vi "Update Library.vi"(8 "error in":errorcluster, 10 "Library":refnum<class "Library.lvclass">, 11 "Project in":refnum<class "Project.lvclass">) -> (0 "error out":errorcluster, 3 "Project out":refnum<class "Project.lvclass">)   [LabVIEW 2020, in "Panther Dashboard.lvlib" / "Project.lvclass"]
uses:
  Project.lvclass
  Library/Library.lvclass
  C:/GitClones/PantherDashboard/src/LabVIEW/Panther Dashboard/Class/LabVIEWItem/LabVIEWItem.lvclass
  Project.lvclass/Project.ctl
  LabVIEWItem/LabVIEWItem.lvclass/LabVIEWItem.ctl
  Library/Library.lvclass/Library.ctl
  Library/Read Library Ref.vi
  Library/Write Library Ref.vi
  LabVIEWItem/Read Item Path.vi
  Read Libraries.vi
  Write Libraries.vi
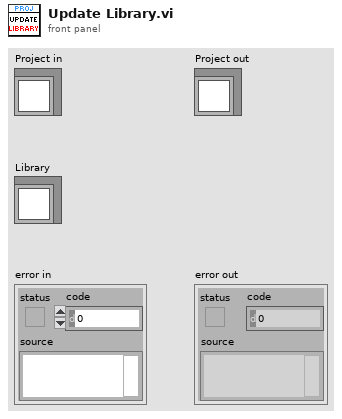
[diagram p1: front panel]
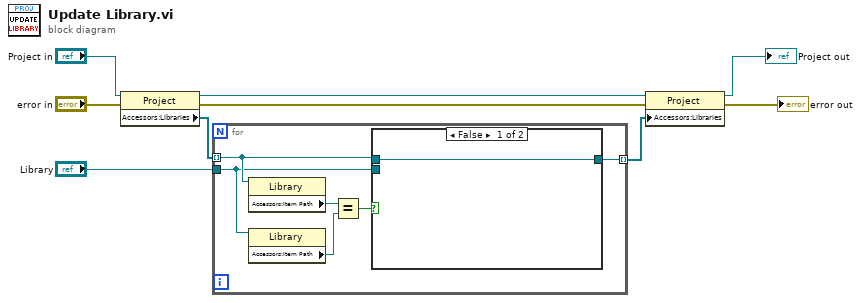
[diagram p0: block diagram]
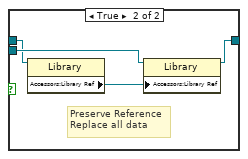
[diagram p2: hidden frame]
diagram:
  n1 = property class="Project"(reference="Project in", error in="error in") -> (reference out=w4:refnum<class "Project.lvclass">, error out=w8:errorcluster, "Accessors:Libraries"=w5:refnum<class "Library.lvclass">[])
  n2 = for {
    tunnel: w5 -> [w12] mode=indexing
    tunnel: [w11] -> w2 mode=indexing
    tunnel: "Library" -> [w10]
    n3 = property class="Library"(reference=w12) -> ("Accessors:Item Path"=w15:path)  [unwired: 1 in, 2 out]
    n4 = property class="Library"(reference=w10) -> ("Accessors:Item Path"=w14:path)  [unwired: 1 in, 2 out]
    n5 = Equal?(x=w15, y=w14) -> (x = y?=w13:bool)
    n6 = case shown="False" w13 {
      tunnel: w12 -> [w16 w19]
      tunnel: [w16 w18] -> w11
      tunnel: w10 -> [_ w20]
      frame False {
      }
      frame True {
        # "Preserve Reference\nReplace all data"
        n7 = property class="Library"(reference=w19) -> ("Accessors:Library Ref"=w17:refnum<vi>)  [unwired: 1 in, 2 out]
        n8 = property class="Library"(reference=w20, "Accessors:Library Ref"=w17) -> (reference out=w18:refnum<class "Library.lvclass">)  [unwired: 1 in, 1 out]
      }
    }
  }
  n9 = property class="Project"(reference=w4, error in=w8, "Accessors:Libraries"=w2) -> (reference out=→"Project out":refnum<class "Project.lvclass">, error out=→"error out":errorcluster)
